vi "OAT Get Slow Roll Vectors (1 Channel).vi"(0 "scaled signal [EU]":waveform(dbl)={"t0"=timestamp(0 s since 1904-01-01), "dt"=0.0, "Y"=[]}, 1 "reference output mode":T1(ring), 2 "reset? (T)":bool=TRUE, 5 "speed profile":T2 {"speed [RPM]" format="%.2f"; "time [s]" format="%.2f"}, 7 "pulse/revolution (1)":i32=1, 9 "orders to compensate (1.0)":dbl[](array[numeric])=[1.0] format="%.2f", 11 "error in (no error)":errorcluster, 12 "bandwidth [order]":dbl format="%.2f") -> (4 "vector references":cdb[](array[numeric]) format="%.2f", 15 "error out":errorcluster)   [LabVIEW 2017]
uses:
  <vilib>/addons/Sound and Vibration/Order Analysis/Tach Process/SubVIs/speed profile.ctl
  <vilib>/addons/Sound and Vibration/Order Analysis/Resample Order Tracking/OAT Order Magnitude and Phase (Even Angle Signal, 1 Channel).vi
  <vilib>/addons/Sound and Vibration/Order Analysis/Resample Order Tracking/OAT Convert to Even Angle Signal (1 Channel).vi
  <vilib>/Analysis/NI_AALPro.lvlib
  <vilib>/addons/Sound and Vibration/Order Analysis/Resample Order Tracking/SoundVib_OrderTracking.lvlib
  <vilib>/addons/Sound and Vibration/Order Analysis/Tach Process/SoundVib_TachProcess.lvlib
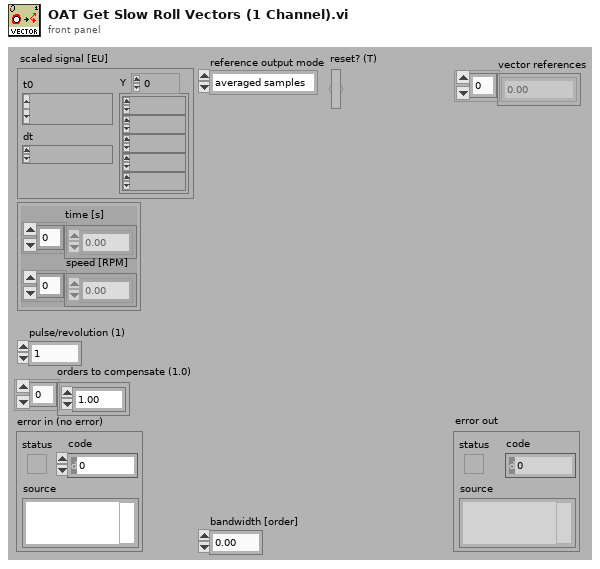
[diagram p1: front panel]
types:
  T1 = enum16{"averaged samples", "initial samples", "final samples"}
  T2 = typedef "SoundVib_TachProcess.lvlib/speed profile.ctl" = cluster{"time [s]":dbl[], "speed [RPM]":dbl[]}
  T3 = cluster{"dB on? (T)":bool, "unwrap phase? (T)":bool, "unit in degree? (T)":bool}
  T4 = typedef "svc_Resampled Channel Info.ctl" = cluster{"channel name":string, "description":string, " channel info":T5}
  T5 = typedef "svc_Channel Info.ctl" = cluster{"sensor sensitivity":dbl, "engineering units":T6, "dB reference":dbl, "custom label":string, "weighting filter":T7, "pregain":dbl}
  T6 = typedef "svc_Engineering Units Text Ring.ctl" = u16
  T7 = typedef "svc_Weighting Filter Text Ring.ctl" = u16
  T8 = typedef "OAT Position Info.ctl" = cluster{"positions [s]":dbl[], "samples/rev":dbl}
  T9 = cluster{"time/rev/rpm":dbl[], "magnitude":dbl[]}[]
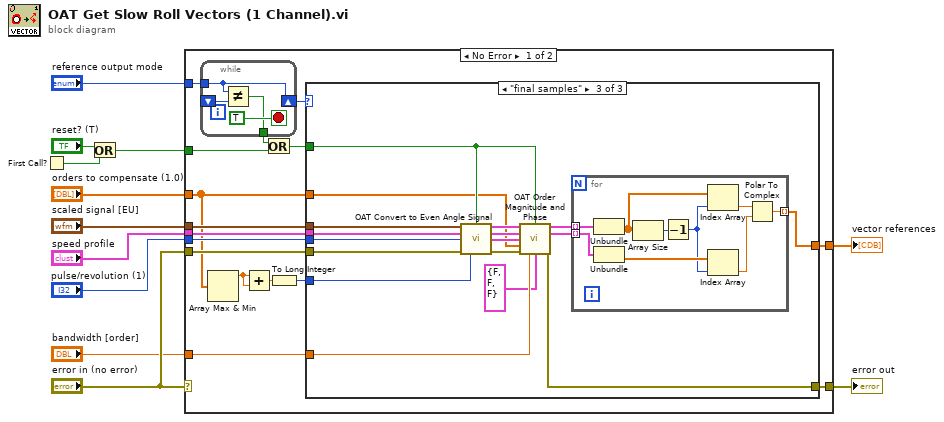
[diagram p0: block diagram]
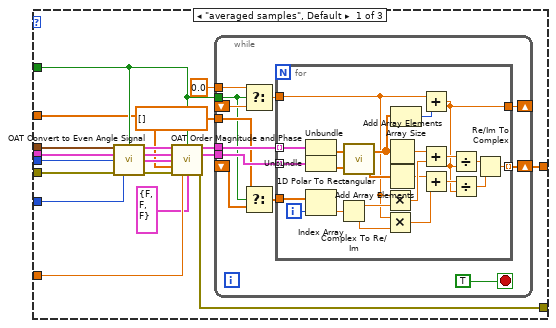
[diagram p2: hidden frame]
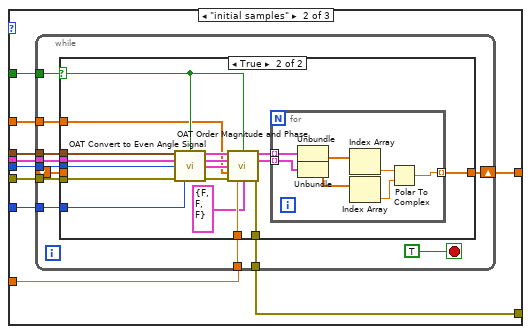
[diagram p3: hidden frame]
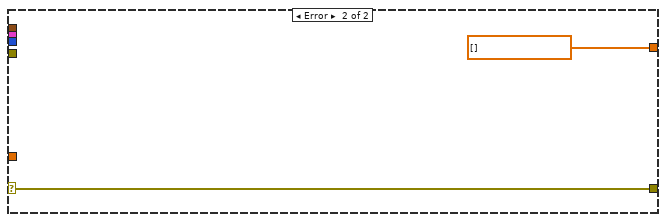
[diagram p5: hidden frame]
diagram:
  n1 = First Call?() -> (First Call?: T/F=w5:bool)
  n2 = Or(x="reset? (T)", y=w5) -> (x .or. y?=w4:bool)
  n3 = case shown="No Error" "error in (no error)" {
    selector: "error in (no error)" -> [_ w161]
    tunnel: "scaled signal [EU]" -> [w22 _]
    tunnel: "speed profile" -> [w28 _]
    tunnel: "pulse/revolution (1)" -> [w27 _]
    tunnel: "error in (no error)" -> [w26 _]
    tunnel: [w25 cdb[] []] -> w8
    tunnel: [w24 w161] -> w7
    tunnel: w4 -> [w18 _]
    tunnel: "bandwidth [order]" -> [w23 _]
    tunnel: "orders to compensate (1.0)" -> [w14 _]
    tunnel: "reference output mode" -> [w21 _]
    frame No Error {
      n4 = while {
        shift-right: [w32] -> w20
        shift-left: _ -> [w31]
        tunnel: w21 -> [w32]
        tunnel: [w29] -> w19
        stop <- TRUE stop-if-true
        n5 = Not Equal?(x=w32, y=w31) -> (x != y?=w29:bool)
      }
      n6 = Array Max & Min(array=w14) -> (max value=w15:dbl)  [unwired: 3 out]
      n7 = Add(x=w15, y=w15) -> (x+y=w16:dbl)
      n8 = Or(x=w19, y=w18) -> (x .or. y?=w17:bool)
      n9 = To Long Integer(number=w16) -> (32bit integer=w13:i32)
      n10 = case shown="\"final samples\"" w20 {
        tunnel: w22 -> [w51 w96 w151]
        tunnel: w28 -> [w50 w95 w150]
        tunnel: w27 -> [w49 w94 w149]
        tunnel: w26 -> [w48 w93 w148]
        tunnel: [w39 w92 w147] -> w25
        tunnel: [w41 w91 w146] -> w24
        tunnel: w23 -> [w40 w90 w145]
        tunnel: w14 -> [w35 w89 w137]
        tunnel: w17 -> [w36 w88 w138]
        tunnel: w13 -> [w34 w87 w136]
        frame "averaged samples", Default {
          n11 = call-poly <vilib>:"OAT Convert to Even Angle Signal.vi"("scaled signal [EU]"=w51, "reset? (F)"=w36, "speed profile"=w50, "pulse/revolution (1)"=w49, "error in (no error)"=w48, "max order (auto)"=w34) -> ("even-angle signal"=w47:cluster{"r0":dbl, "dr":dbl, "Y":dbl[]}, "even-angle channel info"=w46:T4, "even-angle position info"=w45:T8, "error out"=w44:errorcluster)  [unwired: 5 in, 1 out]
          n12 = call-poly <vilib>:"OAT Order Magnitude and Phase.vi"("even-angle signal"=w47, "reset? (F)"=w36, "even-angle channel info"=w46, "even-angle position info"=w45, "orders to compute (1.0)"=w35, "error in (no error)"=w44, "bandwidth [order]"=w40, "view"=T3 {"dB on? (T)"=FALSE, "unwrap phase? (T)"=FALSE, "unit in degree? (T)"=FALSE}) -> ("magnitudes [RMS]"=w43:T9, "phases [phase lag]"=w42:cluster{"time/rev/rpm":dbl[], "phase":dbl[]}[], "error out"=w41:errorcluster)  [unwired: 2 in, 3 out]
          n13 = while {
            tunnel: w43 -> [w63]
            tunnel: w42 -> [w62]
            shift-right: [w59] -> _
            shift-left: _ -> [w58]
            shift-right: [w60] -> w39
            shift-left: _ -> [w56]
            tunnel: w36 -> [w53]
            tunnel: 0.0 -> [w55]
            tunnel: cdb[] [] -> [w54]
            stop <- TRUE stop-if-true
            n14 = Select(t=w55, s=w53, f=w58) -> (s? t:f=w57:dbl)
            n15 = Select(t=w54, s=w53, f=w56) -> (s? t:f=w52:cdb[])
            n16 = for {
              tunnel: w63 -> [w86] mode=indexing
              tunnel: w62 -> [w85] mode=indexing
              tunnel: [w83] -> w60 mode=indexing
              tunnel: [w70] -> w59
              tunnel: w57 -> [w64]
              tunnel: w52 -> [w67]
              i -> [w65]
              n17 = Unbundle(w86) -> ("magnitude"=w84:dbl[])  [unwired: 1 out]
              n18 = Unbundle(w85) -> ("phase"=w82:dbl[])  [unwired: 1 out]
              n19 = Index Array(array=w67, index=w65) -> (element=w66:cdb)
              n20 = Complex To Re/Im(x + iy=w66) -> (x=w80:dbl, y=w79:dbl)
              n21 = call <vilib>:"1D Polar To Rectangular.vi"("Magnitude"=w84, "Phase"=w82) -> ("X"=w78:dbl[], "Y"=w77:dbl[])  [unwired: 1 out]
              n22 = Multiply(x=w64, y=w80) -> (x*y=w75:dbl)
              n23 = Multiply(x=w64, y=w79) -> (x*y=w73:dbl)
              n24 = Add Array Elements(numeric array=w78) -> (sum=w76:dbl)
              n25 = Add Array Elements(numeric array=w77) -> (sum=w74:dbl)
              n26 = Array Size(array=w78) -> (size(s)=w81:i32)
              n27 = Add(x=w64, y=w81) -> (x+y=w70:dbl)
              n28 = Add(x=w76, y=w75) -> (x+y=w72:dbl)
              n29 = Add(x=w74, y=w73) -> (x+y=w71:dbl)
              n30 = Divide(x=w72, y=w70) -> (x/y=w69:dbl)
              n31 = Divide(x=w71, y=w70) -> (x/y=w68:dbl)
              n32 = Re/Im To Complex(1:w68, 2:w69) -> (0:w83:cdb)
            }
          }
        }
        frame "initial samples" {
          n33 = while {
            tunnel: w96 -> [w108]
            tunnel: w95 -> [w107]
            tunnel: w94 -> [w106]
            tunnel: w93 -> [w105]
            tunnel: [w103] -> w91
            tunnel: w90 -> [w102]
            tunnel: w89 -> [w98]
            tunnel: w88 -> [w101]
            shift-right: [w104] -> w92
            shift-left: _ -> [w99]
            tunnel: w87 -> [w97]
            stop <- TRUE stop-if-true
            n34 = case shown="True" w101 {
              selector: w101 -> [_ w114]
              tunnel: w108 -> [_ w127]
              tunnel: w107 -> [_ w126]
              tunnel: w106 -> [_ w125]
              tunnel: w105 -> [w110 w124]
              tunnel: [w109 w117] -> w104
              tunnel: [w110 w116] -> w103
              tunnel: w102 -> [_ w115]
              tunnel: w99 -> [w109 _]
              tunnel: w98 -> [_ w113]
              tunnel: w97 -> [_ w112]
              frame False {
              }
              frame True {
                n35 = call-poly <vilib>:"OAT Convert to Even Angle Signal.vi"("scaled signal [EU]"=w127, "reset? (F)"=w114, "speed profile"=w126, "pulse/revolution (1)"=w125, "error in (no error)"=w124, "max order (auto)"=w112) -> ("even-angle signal"=w123:cluster{"r0":dbl, "dr":dbl, "Y":dbl[]}, "even-angle channel info"=w122:T4, "even-angle position info"=w121:T8, "error out"=w120:errorcluster)  [unwired: 5 in, 1 out]
                n36 = call-poly <vilib>:"OAT Order Magnitude and Phase.vi"("even-angle signal"=w123, "reset? (F)"=w114, "even-angle channel info"=w122, "even-angle position info"=w121, "orders to compute (1.0)"=w113, "error in (no error)"=w120, "bandwidth [order]"=w115, "view"=T3 {"dB on? (T)"=FALSE, "unwrap phase? (T)"=FALSE, "unit in degree? (T)"=FALSE}) -> ("magnitudes [RMS]"=w119:T9, "phases [phase lag]"=w118:cluster{"time/rev/rpm":dbl[], "phase":dbl[]}[], "error out"=w116:errorcluster)  [unwired: 2 in, 3 out]
                n37 = for {
                  tunnel: w119 -> [w134] mode=indexing
                  tunnel: w118 -> [w133] mode=indexing
                  tunnel: [w128] -> w117 mode=indexing
                  n38 = Unbundle(w134) -> ("magnitude"=w132:dbl[])  [unwired: 1 out]
                  n39 = Unbundle(w133) -> ("phase"=w131:dbl[])  [unwired: 1 out]
                  n40 = Index Array(array=w132) -> (element=w130:dbl)  [unwired: 1 in]
                  n41 = Index Array(array=w131) -> (element=w129:dbl)  [unwired: 1 in]
                  n42 = Polar To Complex(1:w129, 2:w130) -> (0:w128:cdb)
                }
              }
            }
          }
        }
        frame "final samples" {
          n43 = call-poly <vilib>:"OAT Convert to Even Angle Signal.vi"("scaled signal [EU]"=w151, "reset? (F)"=w138, "speed profile"=w150, "pulse/revolution (1)"=w149, "error in (no error)"=w148, "max order (auto)"=w136) -> ("even-angle signal"=w144:cluster{"r0":dbl, "dr":dbl, "Y":dbl[]}, "even-angle channel info"=w143:T4, "even-angle position info"=w142:T8, "error out"=w141:errorcluster)  [unwired: 5 in, 1 out]
          n44 = call-poly <vilib>:"OAT Order Magnitude and Phase.vi"("even-angle signal"=w144, "reset? (F)"=w138, "even-angle channel info"=w143, "even-angle position info"=w142, "orders to compute (1.0)"=w137, "error in (no error)"=w141, "bandwidth [order]"=w145, "view"=T3 {"dB on? (T)"=FALSE, "unwrap phase? (T)"=FALSE, "unit in degree? (T)"=FALSE}) -> ("magnitudes [RMS]"=w140:T9, "phases [phase lag]"=w139:cluster{"time/rev/rpm":dbl[], "phase":dbl[]}[], "error out"=w146:errorcluster)  [unwired: 2 in, 3 out]
          n45 = for {
            tunnel: w140 -> [w160] mode=indexing
            tunnel: w139 -> [w159] mode=indexing
            tunnel: [w155] -> w147 mode=indexing
            n46 = Unbundle(w160) -> ("magnitude"=w154:dbl[])  [unwired: 1 out]
            n47 = Unbundle(w159) -> ("phase"=w158:dbl[])  [unwired: 1 out]
            n48 = Array Size(array=w154) -> (size(s)=w153:i32)
            n49 = Decrement(x=w153) -> (x-1=w152:i32)
            n50 = Index Array(array=w154, index=w152) -> (element=w157:dbl)
            n51 = Index Array(array=w158, index=w152) -> (element=w156:dbl)
            n52 = Polar To Complex(1:w156, 2:w157) -> (0:w155:cdb)
          }
        }
      }
    }
    frame Error {
    }
  }
  "error out" <- w7
  "vector references" <- w8
